vi "Create Folder If DNE.vi"(8 "Error In":errorcluster, 11 "Folder Path":path) -> (0 "Error Out":errorcluster, 3 "Dup Path":path)   [LabVIEW 2011, in "LVH-Toolbox.lvlib" / "LVH-Build-Tools.lvlib"]
uses:
  Build Tools/LVH-Build-Tools.lvlib
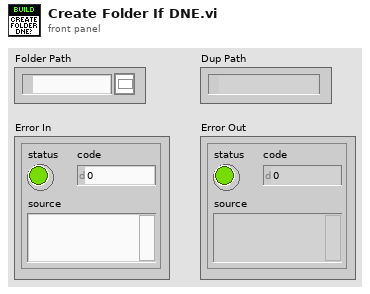
[diagram p1: front panel]
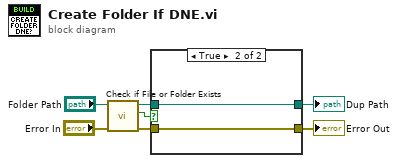
[diagram p0: block diagram]
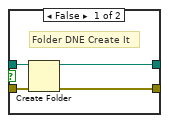
[diagram p2: hidden frame]
diagram:
  n1 = call <vilib>:"Check if File or Folder Exists.vi"("error in (no error)"="Error In", "path"="Folder Path") -> ("error out"=w2:errorcluster, "file or folder exists?"=w3:bool, "dup path"=w4:path)  [unwired: 7 in]
  n2 = case shown="True" w3 {
    tunnel: [w9 w13] -> w5
    tunnel: w2 -> [w11 w13]
    tunnel: w4 -> [w10 w12]
    tunnel: [w8 w12] -> w7
    frame False {
      # "Folder DNE Create It"
      n3 = Create Folder(path (use dialog)=w10, error in=w11) -> (created path=w8:path, error out=w9:errorcluster)  [unwired: 1 in, 1 out]
    }
    frame True {
    }
  }
  "Dup Path" <- w7
  "Error Out" <- w5
